vi "Update Target SV Tree.vi"(7 "TreeControl in":refnum<vi>, 8 "error in (no error)":errorcluster, 11 "Variable list compared":refnum<class "ChannelVS.lvclass">[](array[class])) -> (0 "error out":errorcluster)   [LabVIEW 2017, in "Shared Variables CD 2.0 Configuration.lvlib"]
uses:
  Shared Variables CD 2.0 Configuration.lvlib
  ChannelVS/ChannelVS.lvclass
  ChannelVS/ChannelVS.lvclass/ChannelVS.ctl
  Public/Documents/National Instruments/NI VeriStand 2017/Custom Devices/Shared Variables CD 2.0/Data/Channel.lvlibp/Channel.lvclass
  C:/Users/Public/Documents/National Instruments/NI VeriStand 2017/Custom Devices/Shared Variables CD 2.0/Data/Channel.lvlibp/Channel.lvclass
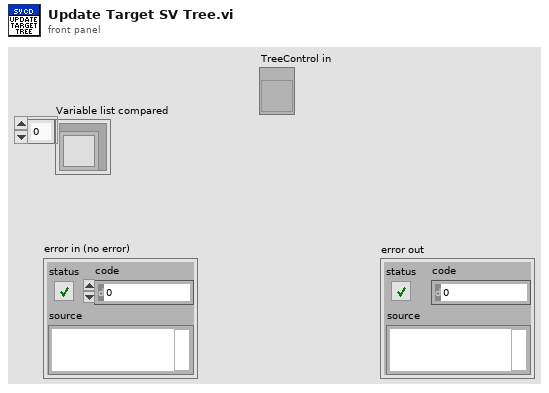
[diagram p1: front panel]
types:
  T1 = typedef "Channel.lvlibp/NI_Data Type.lvlib/Data Type.ctl" = enum8{"Invalid Type", "Void", "I8", "I16", "I32", "I64", "U8", "U16", "U32", "U64", "Single Float", "Double Float", "Extended Float", "Single Complex", "Double Complex", "Extended Complex", "Enum U8", "Enum U16", "Enum U32", "Enum U64", "Single Float With Unit", "Double Float With Unit", "Extended Float With Unit", "Single Complex with Unit", "Double Complex with Unit", "Extended Complex with Unit", "Boolean", "String", "Path", "Picture", "Tag", "Array", "Cluster", "Variant", "LV Variant", "Waveform", "Timestamp", "Digital Waveform", "Digital Data", "ExpressData", "Refnum", "External Data", "VI", "Poly VI", "LabVIEW Class Instance", "Fixed Point"}
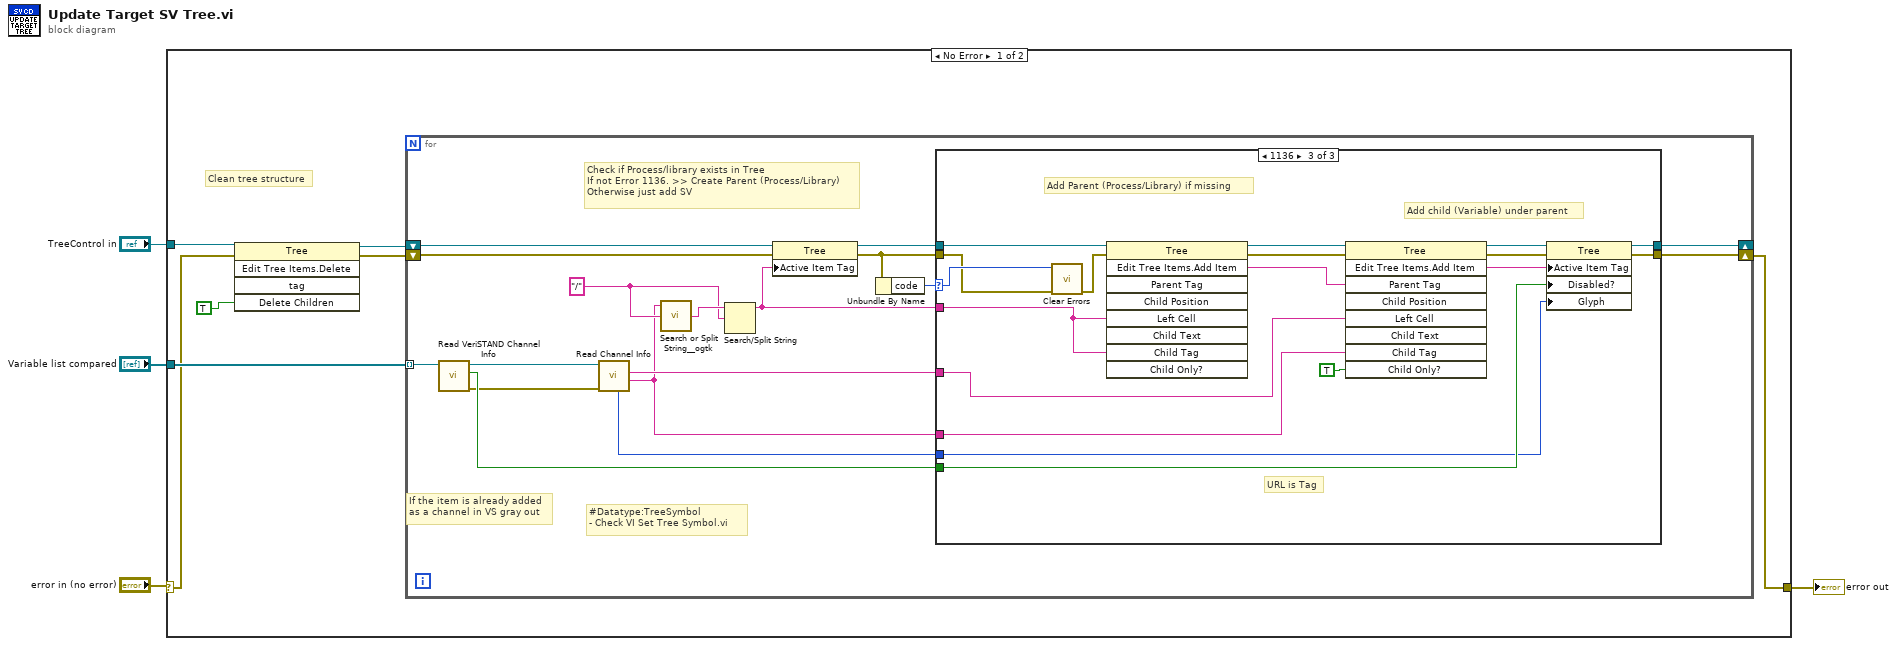
[diagram p0: block diagram]
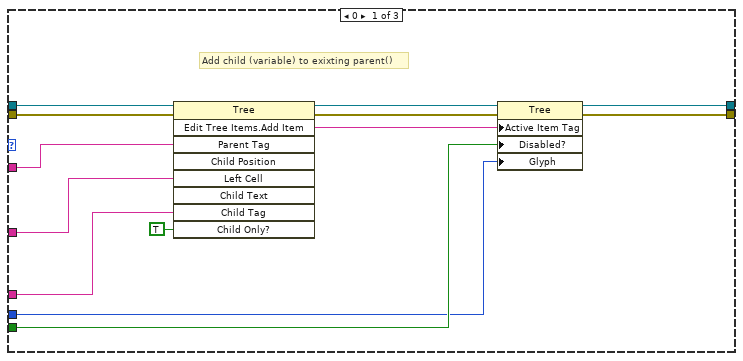
[diagram p2: hidden frame]
diagram:
  n1 = case shown="No Error" "error in (no error)" {
    selector: "error in (no error)" -> [w9 w62]
    tunnel: "TreeControl in" -> [w6 _]
    tunnel: "Variable list compared" -> [w11 _]
    tunnel: [w10 w62] -> w2
    frame No Error {
      # "Clean tree structure"
      n2 = invoke class="Tree" method="Edit Tree Items.Delete"(reference=w6, error in=w9, "Delete Children"=TRUE ("Delete Children?")) -> (reference out=w7:refnum<vi>, error out=w8:errorcluster)  [unwired: 2 in, 3 out]
      n3 = for {
        tunnel: w11 -> [w14] mode=indexing
        shift-right: [w20] -> _
        shift-left: w7 -> [w23]
        shift-right: [w19] -> w10
        shift-left: w8 -> [w22]
        w21 = "/" ("search string/char (-)")
        # "If the item is already added\nas a channel in VS gray out"
        # "#Datatype:TreeSymbol\n- Check VI Set Tree Symbol.vi"
        # "Check if Process/library exists in Tree \nIf not Error 1136. >> Create Parent (Process/Library)\nOtherwise just add SV"
        n4 = call "Read VeriSTAND Channel Info.vi"("ChannelVS in"=w14) -> ("error out"=w15:errorcluster, "Exist in VeriSTAND"=w16:bool, "ChannelVS out"=w13:refnum<class "ChannelVS.lvclass">)  [unwired: 7 in, 1 out]
        n5 = call "Read Channel Info.vi"("error in (no error)"=w15, "Channel in"=w13) -> ("URL"=w12:string, "Name"=w18:string, "DataType"=w17:T1)  [unwired: 4 in, 3 out]
        n6 = call <userlib>:"Search or Split String__ogtk.vi"("search string/char (-)"=w21, "string"=w12) -> ("substring after match"=w28:string)  [unwired: 1 in, 2 out]
        n7 = Search/Split String(string=w28, search string/char (-)=w21) -> (substring before match=w24:string)  [unwired: 1 in, 2 out]
        n8 = property class="Tree"(reference=w23, error in=w22, "Active Item Tag"=w24) -> (reference out=w26:refnum<vi>, error out=w25:errorcluster)
        n9 = Unbundle By Name(w25) -> ("code"=w27:i32)
        n10 = case shown="1136" w27 {
          selector: w27 -> [_ _ w56]
          tunnel: w12 -> [w35 _ w52]
          tunnel: w24 -> [w41 _ w60]
          tunnel: w26 -> [w40 w43 w61]
          tunnel: w25 -> [w39 w42 w55]
          tunnel: [w33 w42 w48] -> w19
          tunnel: [w34 w43 w50] -> w20
          tunnel: w18 -> [w38 _ w53]
          tunnel: w16 -> [w31 _ w46]
          tunnel: w17 -> [w30 _ w45]
          frame 0 {
            # "Add child (variable) to exixting parent()"
            n11 = invoke on="Invoke Node" class="Tree" method="Edit Tree Items.Add Item"(reference=w40, error in=w39, "Parent Tag"=w41, "Left Cell"=w38, "Child Tag"=w35, "Child Only?"=TRUE) -> (reference out=w37:refnum<vi>, error out=w36:errorcluster, "Edit Tree Items:Add Item"=w29:string)  [unwired: 3 in, 6 out]
            n12 = property class="Tree"(reference=w37, error in=w36, "Active Item Tag"=w29, "Disabled?"=w31, "Glyph"=w30) -> (reference out=w34:refnum<vi>, error out=w33:errorcluster)
          }
          frame Default {
          }
          frame 1136 {
            # "Add child (Variable) under parent"
            # "Add Parent (Process/Library) if missing"
            # "URL is Tag"
            n13 = call <vilib>:"Clear Errors.vi"("error in (no error)"=w55, "specific error code to clear (0: all)"=w56) -> ("error out"=w54:errorcluster)  [unwired: 4 in, 1 out]
            n14 = invoke class="Tree" method="Edit Tree Items.Add Item"(reference=w61, error in=w54, "Left Cell"=w60, "Child Tag"=w60) -> (reference out=w59:refnum<vi>, error out=w58:errorcluster, "Edit Tree Items:Add Item"=w57:string)  [unwired: 5 in, 6 out]
            n15 = invoke on="Invoke Node" class="Tree" method="Edit Tree Items.Add Item"(reference=w59, error in=w58, "Parent Tag"=w57, "Left Cell"=w53, "Child Tag"=w52, "Child Only?"=TRUE) -> (reference out=w51:refnum<vi>, error out=w49:errorcluster, "Edit Tree Items:Add Item"=w44:string)  [unwired: 3 in, 6 out]
            n16 = property class="Tree"(reference=w51, error in=w49, "Active Item Tag"=w44, "Disabled?"=w46, "Glyph"=w45) -> (reference out=w50:refnum<vi>, error out=w48:errorcluster)
          }
        }
      }
    }
    frame Error {
    }
  }
  "error out" <- w2
